vi "AO Set.vi"(7 "Box ID":u8, 8 "error in (no error)":errorcluster, 9 "AO2 Voltage":dbl min=0.0 max=5.0, 10 "AO1 Voltage":dbl min=0.0 max=5.0, 11 "ENET in":refnum<class "ENET_BS120x.lvclass">) -> (0 "error out":errorcluster, 3 "ENET out":refnum<class "ENET_BS120x.lvclass">)   [LabVIEW 2021, in "BS120x Driver.lvlib" / "ENET_BS120x.lvclass"]
uses:
  ENET_BS120x.lvclass
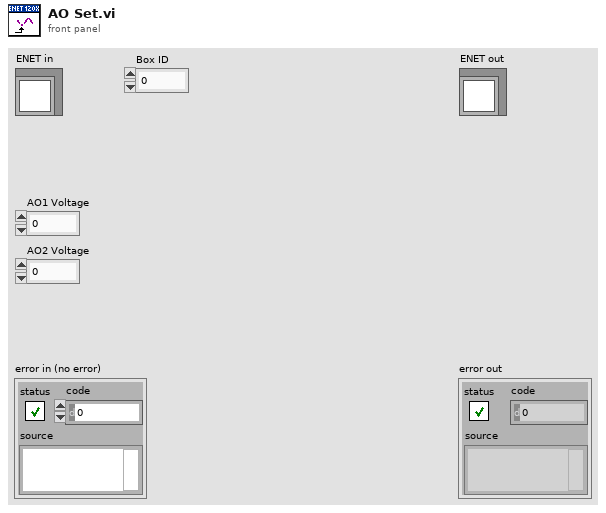
[diagram p1: front panel]
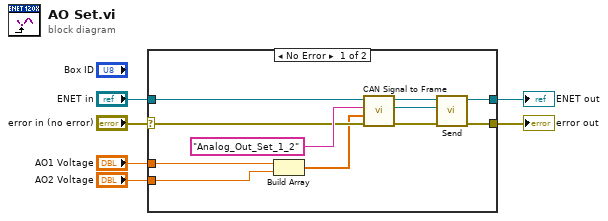
[diagram p0: block diagram]
diagram:
  n1 = case shown="No Error" "error in (no error)" {
    selector: "error in (no error)" -> [w10 w18]
    tunnel: [w13 w18] -> w6
    tunnel: "AO1 Voltage" -> [w12 _]
    tunnel: "AO2 Voltage" -> [w11 _]
    tunnel: "ENET in" -> [w8 w19]
    tunnel: [w7 w19] -> w1
    frame No Error {
      n2 = Build Array(w12, w11) -> (w9:dbl[])
      n3 = call "CAN Signal to Frame.vi"("error in (no error)"=w10, "Data Array"=w9, "Frame"="Analog_Out_Set_1_2", "ENET in"=w8) -> ("error out"=w14:errorcluster, "Data"=w15:refnum<class "Data.lvclass">, "ENET out"=w16:refnum<class "ENET_BS120x.lvclass">)  [unwired: 5 in]
      n4 = call "Send.vi"("error in (no error)"=w14, "Data"=w15, "ENET in"=w16) -> ("error out"=w13:errorcluster, "ENET out"=w7:refnum<class "ENET_BS120x.lvclass">)  [unwired: 7 in]
    }
    frame Error {
    }
  }
  "error out" <- w6
  "ENET out" <- w1
